vi "_UtilsRandomBoolValue.vi"(1 "factor":dbl=1.0) -> (0 "random value":bool)   [LabVIEW 2014, in "examples.lvlib"]
uses:
  examples.lvlib
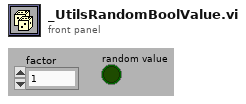
[diagram p1: front panel]
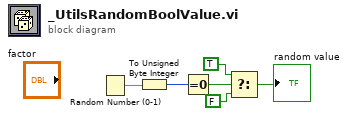
[diagram p0: block diagram]
diagram:
  n1 = Random Number (0-1)() -> (number: 0 to 1=w6:dbl)
  n2 = To Unsigned Byte Integer(number=w6) -> (unsigned 8bit integer=w5:u8)
  n3 = Equal To 0?(x=w5) -> (x = 0?=w4:bool)
  n4 = Select(t=TRUE, s=w4, f=FALSE) -> (s? t:f=→"random value":bool)
